vi "Find Top Level core.vi"(8 "error in (no error)":errorcluster, 10 "VI":string, 11 "Panel Registry in":refnum<class "Panel Registry.lvclass">) -> (0 "error out":errorcluster, 1 "Found?":bool, 2 "Top Level Panel":string)   [LabVIEW 2023, in "Panel Actor.lvlib" / "Panel.lvlib" / "Panel Registry.lvclass"]
uses:
  Panel Registry.lvclass
  Panel Registry.lvclass/Panel Registry.ctl
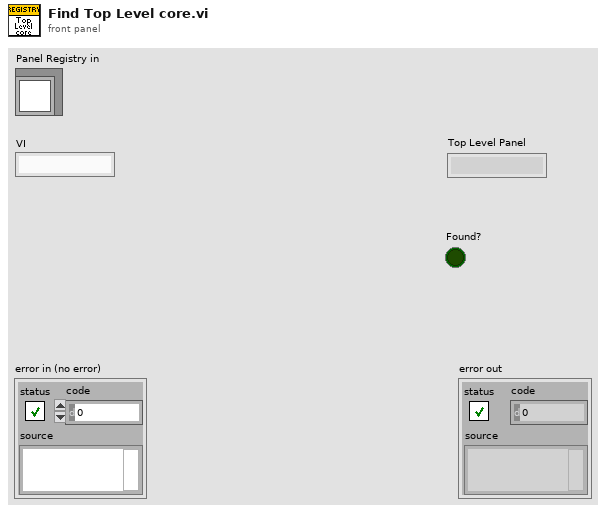
[diagram p1: front panel]
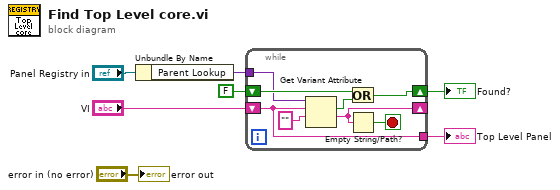
[diagram p0: block diagram]
diagram:
  n1 = Unbundle By Name("Panel Registry in") -> ("Parent Lookup"=w2:variant)
  n2 = while {
    shift-right: [w9] -> _
    shift-left: "VI" -> [w11]
    tunnel: [w11] -> w5
    shift-right: [w14] -> w4
    shift-left: FALSE ("Found?") -> [w13]
    tunnel: w2 -> [w12]
    stop <- w15 stop-if-true
    n3 = Get Variant Attribute(Variant=w12, name=w11, default value (empty Variant)="" ("VI")) -> (found=w8:bool, value=w9:string)  [unwired: 1 in, 2 out]
    n4 = Or(x=w13, y=w8) -> (x .or. y?=w14:bool)
    n5 = Empty String/Path?(string/path=w9) -> (empty?=w15:bool)
  }
  "Top Level Panel" <- w5
  "Found?" <- w4
  "error out" <- "error in (no error)"
